vi "log analysis_gps.vi"() -> ()   [LabVIEW 2019] (continued)
11.969600\t-0.937959\t-0.544053\t72.586704\t0.097000\t0.019000\n\t\n15:28:30.8\tlog_raw\tgps_raw\t\tsystem status\texception 0 28.000000 0 60\trobot status\t346.259723\t26.589549\t11.968800\t-0.938206\t-0.546014\t72.587898\t0.097000\t0.019000\n\t\n15:28:31.3\tlog_raw\tgps_raw\t\tsystem status\texception 0 28.100000 0 60\trobot status\t346.261225\t26.595016\t11.967900\t-0.938058\t-0.546498\t72.587416\t0.097000\t0.019000\n\t\n15:28:31.8\tlog_raw\tgps_raw\t\tsystem status\texception 0 28.100000 0 60\trobot status\t346.263217\t26.600750\t11.967200\t-0.937314\t-0.548987\t72.586839\t0.097000\t0.019000\n\t\n15:28:32.3\tlog_raw\tgps_raw\t\tsystem status\texception 0 28.100000 0 60\trobot status\t346.266027\t26.606616\t11.967100\t-0.934688\t-0.548051\t72.585281\t0.097000\t0.019000\n\t\n15:28:32.8\tlog_raw\tgps_raw\t\tsystem status\texception 0 28.000000 0 60\trobot status\t346.269388\t26.612663\t11.967500\t-0.933167\t-0.552134\t72.585486\t0.097000\t0.019000\n\t\n15:28:33.3\tlog_raw\tgps_raw\t\tsystem status\texception 0 28.100000 0 60\trobot status\t346.272370\t26.617656\t11.968500\t-0.933128\t-0.553139\t72.580572\t0.097000\t0.019000\n\t\n15:28:33.8\tlog_raw\tgps_raw\t\tsystem status\texception 0 28.000000 0 60\trobot status\t346.274708\t26.622212\t11.969900\t-0.932001\t-0.554064\t72.578346\t0.097000\t0.019000\n\t\n15:28:34.3\tlog_raw\tgps_raw\t\tsystem status\texception 0 28.000000 0 60\trobot status\t346.272071\t26.616055\t11.970100\t-0.930607\t-0.553691\t72.568592\t0.097000\t0.019000\n\t\n15:28:34.8\tlog_raw\tgps_raw\t#INSPVAXA,USB3,0,50.0,FINESTEERING,2107,282532.800,02000000,471d,15824;INS_ALIGNMENT_COMPLETE,INS_RTKFIXED,37.37036990032,126.72474422565,11.9691,22.3000,0.0075,0.0051,0.0018,-0.932116001,-0.549055451,17.452522918,0.2503,0.2036,0.3279,0.0447,0.0435,0.0399,0.0917,0.0916,4.9913,0f000005,0*47d3a519\n\tsystem status\texception 0 28.000000 0 60\trobot status\t346.263495\t26.596260\t11.969100\t-0.932116\t-0.549055\t72.547477\t0.097000\t0.019000\n\t\n15:28:35.3\tlog_raw\tgps_raw\t\tsystem status\texception 0 28.000000 0 60\trobot status\t346.259446\t26.587060\t11.968800\t-0.932260\t-0.546298\t72.538547\t0.097000\t0.019000\n\t\n15:28:35.8\tlog_raw\tgps_raw\t\tsystem status\texception 0 28.000000 0 60\trobot status\t346.258585\t26.585056\t11.968900\t-0.932112\t-0.548446\t72.536891\t0.097000\t0.019000\n\t\n15:28:36.3\tlog_raw\tgps_raw\t\tsystem status\texception 0 28.000000 0 60\trobot status\t346.258032\t26.583583\t11.969100\t-0.930409\t-0.549639\t72.534290\t0.097000\t0.019000\n\t\n15:28:36.8\tlog_raw\tgps_raw\t\tsystem status\tnormal 0 28.000000 0 0\trobot status\t346.258148\t26.582748\t11.969400\t-0.931772\t-0.548957\t72.530403\t0.000000\t0.000000\n\t\n15:28:37.3\tlog_raw\tgps_raw\t\tsystem status\tnormal 0 28.100000 0 0\trobot status\t346.258252\t26.582082\t11.969800\t-0.931421\t-0.548856\t72.527417\t0.000000\t0.000000\n\t\n15:28:37.8\tlog_raw\tgps_raw\t#INSPVAXA,USB3,0,51.5,FINESTEERING,2107,282535.800,02000000,471d,15824;INS_ALIGNMENT_COMPLETE,INS_RTKFIXED,37.37036976834,126.72474416785,11.9702,22.3000,0.0056,0.0032,0.0025,-0.929895775,-0.548968401,17.475093869,0.2332,0.1853,0.3065,0.0346,0.0344,0.0316,0.0907,0.0908,4.9937,0f000005,0*4023dcd5\n\tsystem status\tnormal 0 28.000000 0 0\trobot status\t346.258376\t26.581613\t11.970200\t-0.929896\t-0.548968\t72.524906\t0.000000\t0.000000\n\t\n15:28:38.3\tlog_raw\tgps_raw\t\tsystem status\tnormal 0 28.100000 0 0\trobot status\t346.258500\t26.581480\t11.970500\t-0.929563\t-0.547939\t72.523200\t0.000000\t0.000000\n\t\n15:28:38.8\tlog_raw\tgps_raw\t\tsystem status\tnormal 0 28.100000 0 0\trobot status\t346.259099\t26.581501\t11.970800\t-0.929146\t-0.547594\t72.520945\t0.000000\t0.000000\n\t\n15:28:39.3\tlog_raw\tgps_raw\t\tsystem status\tnormal 0 28.100000 0 0\trobot status\t346.259649\t26.581507\t11.971100\t-0.930249\t-0.547598\t72.515508\t0.000000\t0.000000\n\t\n15:28:39.8\tlog_raw\tgps_raw\t\tsystem status\tnormal 0 28.000000 0 0\trobot status\t346.260387\t26.581691\t11.971500\t-0.931613\t-0.550759\t72.514164\t0.000000\t0.000000\n\t\n15:28:40.3\tlog_raw\tgps_raw\t\tsystem status\tnormal 0 28.000000 0 0\trobot status\t346.261018\t26.582062\t11.972200\t-0.929740\t-0.553791\t72.508433\t0.000000\t0.000000\n\t\n15:28:40.8\tlog_raw\tgps_raw\t\tsystem status\tnormal 0 28.100000 0 0\trobot status\t346.261462\t26.582894\t11.973100\t-0.928845\t-0.555133\t72.506321\t0.000000\t0.000000\n\t\n15:28:41.3\tlog_raw\tgps_raw\t#INSPVAXA,USB3,0,50.0,FINESTEERING,2107,282539.300,02000000,471d,15824;INS_ALIGNMENT_COMPLETE,INS_RTKFIXED,37.37036978494,126.72474420325,11.9738,22.3000,0.0064,0.0050,0.0000,-0.929010849,-0.553956795,17.498282096,0.2195,0.1742,0.2911,0.0344,0.0343,0.0312,0.0907,0.0907,4.9970,0f000005,0*d5ca5fec\n\tsystem status\tnormal 0 28.000000 0 0\trobot status\t346.261511\t26.583455\t11.973800\t-0.929011\t-0.553957\t72.501718\t0.000000\t0.000000\n\t\n15:28:41.8\tlog_raw\tgps_raw\t#INSPVAXA,USB3,0,50.0,FINESTEERING,2107,282539.800,02000000,471d,15824;INS_ALIGNMENT_COMPLETE,INS_RTKFIXED,37.37036978547,126.72474420294,11.9740,22.3000,0.0057,0.0046,-0.0006,-0.928135353,-0.553814797,17.500957060,0.2195,0.1742,0.2911,0.0344,0.0343,0.0312,0.0907,0.0907,4.9970,0f000005,0*764a2b63\n\tsystem status\tnormal 0 28.000000 0 0\trobot status\t346.261484\t26.583514\t11.974000\t-0.928135\t-0.553815\t72.499043\t0.000000\t0.000000\n\t\n15:28:42.3\tlog_raw\tgps_raw\t\tsystem status\tnormal 0 28.100000 0 0\trobot status\t346.261404\t26.583443\t11.974300\t-0.930384\t-0.553797\t72.496316\t0.000000\t0.000000\n\t\n15:28:42.8\tlog_raw\tgps_raw\t#INSPVAXA,USB3,0,51.5,FINESTEERING,2107,282540.800,02000000,471d,15824;INS_ALIGNMENT_COMPLETE,INS_RTKFIXED,37.37036978786,126.72474420160,11.9749,22.3000,0.0059,0.0033,-0.0010,-0.930808234,-0.552950862,17.507619402,0.2170,0.1726,0.2881,0.0344,0.0343,0.0312,0.0907,0.0907,4.9979,0f000005,0*a62a7559\n\tsystem status\tnormal 0 28.100000 0 0\trobot status\t346.261365\t26.583779\t11.974900\t-0.930808\t-0.552951\t72.492381\t0.000000\t0.000000\n\t\n15:28:43.3\tlog_raw\tgps_raw\t#INSPVAXA,USB3,0,52.0,FINESTEERING,2107,282541.300,02000000,471d,15824;INS_ALIGNMENT_COMPLETE,INS_RTKFIXED,37.37036978965,126.72474419874,11.9755,22.3000,0.0062,0.0033,-0.0009,-0.929974258,-0.549981203,17.509762902,0.2148,0.1713,0.2853,0.0344,0.0343,0.0312,0.0907,0.0906,4.9990,0f000005,0*bfdf10fc\n\tsystem status\tnormal 0 28.000000 0 0\trobot status\t346.261112\t26.583978\t11.975500\t-0.929974\t-0.549981\t72.490237\t0.000000\t0.000000\n\t\n15:28:43.8\tlog_raw\tgps_raw\t\tsystem status\tnormal 0 28.100000 0 0\trobot status\t346.261132\t26.584205\t11.975800\t-0.930744\t-0.550329\t72.489076\t0.000000\t0.000000\n\t\n15:28:44.3\tlog_raw\tgps_raw\t#INSPVAXA,USB3,0,51.0,FINESTEERING,2107,282542.300,02000000,471d,15824;INS_ALIGNMENT_COMPLETE,INS_RTKFIXED,37.37036979234,126.72474420075,11.9765,22.3000,0.0055,0.0042,-0.0011,-0.931303287,-0.550383804,17.513004311,0.2130,0.1703,0.2828,0.0344,0.0343,0.0312,0.0907,0.0906,5.0000,0f000005,0*b690bd46\n\tsystem status\tnormal 0 28.000000 0 0\trobot status\t346.261290\t26.584276\t11.976500\t-0.931303\t-0.550384\t72.486996\t0.000000\t0.000000\n\t\n15:28:44.8\tlog_raw\tgps_raw\t\tsystem status\tnormal 0 28.000000 0 0\trobot status\t346.261465\t26.584112\t11.977300\t-0.929492\t-0.551225\t72.486272\t0.000000\t0.000000\n\t\n15:28:45.3\tlog_raw\tgps_raw\t#INSPVAXA,USB3,0,47.5,FINESTEERING,2107,282543.300,02000000,471d,15824;INS_ALIGNMENT_COMPLETE,INS_RTKFIXED,37.37036978809,126.72474420745,11.9781,22.3000,0.0036,0.0055,-0.0013,-0.931308273,-0.552026668,17.515229582,0.2114,0.1694,0.2805,0.0344,0.0343,0.0312,0.0907,0.0906,5.0009,0f000005,0*ba0ef0aa\n\tsystem status\tnormal 0 28.000000 0 0\trobot status\t346.261883\t26.583805\t11.978100\t-0.931308\t-0.552027\t72.484770\t0.000000\t0.000000\n\t\n15:28:45.8\tlog_raw\tgps_raw\t#INSPVAXA,USB3,0,47.5,FINESTEERING,2107,282543.800,02000000,471d,15824;INS_ALIGNMENT_COMPLETE,INS_RTKFIXED,37.37036978808,126.72474421663,11.9786,22.3000,0.0047,0.0067,-0.0013,-0.928872282,-0.553697903,17.517066797,0.2114,0.1694,0.2805,0.0344,0.0343,0.0312,0.0907,0.0906,5.0009,0f000005,0*82370f01\n\tsystem status\tnormal 0 28.100000 0 0\trobot status\t346.262696\t26.583804\t11.978600\t-0.928872\t-0.553698\t72.482933\t0.000000\t0.000000\n\t\n15:28:46.3\tlog_raw\tgps_raw\t#INSPVAXA,USB3,0,48.0,FINESTEERING,2107,282544.300,02000000,471d,15824;INS_ALIGNMENT_COMPLETE,INS_RTKFIXED,37.37036978718,126.72474422252,11.9791,22.3000,0.0050,0.0075,-0.0009,-0.927752537,-0.554071617,17.520424988,0.2100,0.1688,0.2784,0.0344,0.0343,0.0312,0.0907,0.0906,5.0016,0f000005,0*49ddb25e\n\tsystem status\tnormal 0 28.100000 0 0\trobot status\t346.263218\t26.583704\t11.979100\t-0.927753\t-0.554072\t72.479575\t0.000000\t0.000000\n\t\n15:28:46.8\tlog_raw\tgps_raw\t\tsystem status\tnormal 0 28.100000 0 0\trobot status\t346.263972\t26.583698\t11.979500\t-0.928560\t-0.556020\t72.475289\t0.000000\t0.000000\n\t\n15:28:47.3\tlog_raw\tgps_raw\t#INSPVAXA,USB3,0,53.5,FINESTEERING,2107,282545.300,02000000,471d,15824;INS_ALIGNMENT_COMPLETE,INS_RTKFIXED,37.37036978780,126.72474423597,11.9800,22.3000,0.0057,0.0083,-0.0009,-0.928955270,-0.556659183,17.532369164,0.2088,0.1684,0.2765,0.0344,0.0343,0.0312,0.0907,0.0906,5.0023,0f000005,0*6d6cecb2\n\tsystem status\tnormal 0 28.100000 0 0\trobot status\t346.264409\t26.583772\t11.980000\t-0.928955\t-0.556659\t72.467631\t0.000000\t0.000000\n\t\n15:28:47.8\tlog_raw\tgps_raw\t#INSPVAXA,USB3,0,53.5,FINESTEERING,2107,282545.800,02000000,471d,15824;INS_ALIGNMENT_COMPLETE,INS_RTKFIXED,37.37036979074,126.72474423499,11.9811,22.3000,0.0059,0.0071,-0.0001,-0.929937499,-0.555084001,17.534967514,0.2088,0.1684,0.2765,0.0344,0.0343,0.0312,0.0907,0.0906,5.0023,0f000005,0*3f4b51d6\n\tsystem status\tnormal 0 28.000000 0 0\trobot status\t346.264323\t26.584099\t11.981100\t-0.929937\t-0.555084\t72.465032\t0.000000\t0.000000\n\t\n15:28:48.3\tlog_raw\tgps_raw\t#INSPVAXA,USB3,0,52.0,FINESTEERING,2107,282546.300,02000000,471d,15824;INS_ALIGNMENT_COMPLETE,INS_RTKFIXED,37.37036979075,126.72474423167,11.9818,22.3000,0.0060,0.0065,0.0000,-0.930882375,-0.556370443,17.539693499,0.2078,0.1680,0.2748,0.0344,0.0343,0.0312,0.0907,0.0906,5.0033,0f000005,0*966ea92a\n\tsystem status\tnormal 0 28.100000 0 0\trobot status\t346.264029\t26.584100\t11.981800\t-0.930882\t-0.556370\t72.460307\t0.000000\t0.000000\n\t\n15:28:48.8\tlog_raw\tgps_raw\t#INSPVAXA,USB3,0,52.0,FINESTEERING,2107,282546.800,02000000,471d,15824;INS_ALIGNMENT_COMPLETE,INS_RTKFIXED,37.37036979117,126.72474423599,11.9822,22.3000,0.0059,0.0073,0.0004,-0.930733937,-0.558015059,17.542914656,0.2078,0.1680,0.2748,0.0344,0.0343,0.0312,0.0907,0.0906,5.0033,0f000005,0*c41d3119\n\tsystem status\tnormal 0 28.000000 0 0\trobot status\t346.264411\t26.584146\t11.982200\t-0.930734\t-0.558015\t72.457085\t0.000000\t0.000000\n\t\n15:28:49.3\tlog_raw\tgps_raw\t#INSPVAXA,USB3,0,48.0,FINESTEERING,2107,282547.300,02000000,471d,15824;INS_ALIGNMENT_COMPLETE,INS_RTKFIXED,37.37036978952,126.72474423883,11.9826,22.3000,0.0057,0.0074,0.0003,-0.934085906,-0.556515155,17.545794834,0.2070,0.1677,0.2732,0.0344,0.0343,0.0312,0.0907,0.0906,5.0042,0f000005,0*0a93c56e\n\tsystem status\tnormal 0 28.000000 0 0\trobot status\t346.264663\t26.583963\t11.982600\t-0.934086\t-0.556515\t72.454205\t0.000000\t0.000000\n\t\n15:28:49.8\tlog_raw\tgps_raw\t#INSPVAXA,USB3,0,48.0,FINESTEERING,2107,282547.800,02000000,471d,15824;INS_ALIGNMENT_COMPLETE,INS_RTKFIXED,37.37036979022,126.72474424169,11.9829,22.3000,0.0059,0.0077,0.0009,-0.935404379,-0.556069366,17.549298346,0.2070,0.1677,0.2732,0.0344,0.0343,0.0312,0.0907,0.0906,5.0042,0f000005,0*a5f569c8\n\tsystem status\tnormal 0 28.100000 0 0\trobot status\t346.264916\t26.584041\t11.982900\t-0.935404\t-0.556069\t72.450702\t0.000000\t0.000000\n\t\n15:28:50.3\tlog_raw\tgps_raw\t#INSPVAXA,USB3,0,52.0,FINESTEERING,2107,282548.300,02000000,471d,15824;INS_ALIGNMENT_COMPLETE,INS_RTKFIXED,37.37036979009,126.72474424298,11.9833,22.3000,0.0058,0.0072,0.0008,-0.938145117,-0.556054082,17.551756735,0.2062,0.1674,0.2718,0.0344,0.0343,0.0312,0.0907,0.0906,5.0051,0f000005,0*c2e33c02\n\tsystem status\tnormal 0 28.100000 0 0\trobot status\t346.265030\t26.584027\t11.983300\t-0.938145\t-0.556054\t72.448243\t0.000000\t0.000000\n\t\n15:28:50.8\tlog_raw\tgps_raw\t\tsystem status\tnormal 0 28.100000 0 0\trobot status\t346.265084\t26.584261\t11.983800\t-0.940336\t-0.557104\t72.445963\t0.000000\t0.000000\n\t\n15:28:51.3\tlog_raw\tgps_raw\t#INSPVAXA,USB3,0,50.5,FINESTEERING,2107,282549.300,02000000,471d,15824;INS_ALIGNMENT_COMPLETE,INS_RTKFIXED,37.37036979437,126.72474424171,11.9842,22.3000,0.0072,0.0058,0.0011,-0.941172709,-0.557765925,17.557830544,0.2056,0.1673,0.2705,0.0344,0.0343,0.0312,0.0907,0.0905,5.0063,0f000005,0*401534f2\n\tsystem status\tnormal 0 28.100000 0 0\trobot status\t346.264918\t26.584502\t11.984200\t-0.941173\t-0.557766\t72.442169\t0.000000\t0.000000\n\t\n15:28:51.8\tlog_raw\tgps_raw\t#INSPVAXA,USB3,0,50.5,FINESTEERING,2107,282549.800,02000000,471d,15824;INS_ALIGNMENT_COMPLETE,INS_RTKFIXED,37.37037057498,126.72474454669,11.9842,22.3000,0.3344,0.1212,-0.0021,-0.779908756,-0.829652021,16.234479944,0.2056,0.1673,0.2705,0.0344,0.0343,0.0312,0.0907,0.0905,5.0063,0f000005,0*992e23a9\n\tsystem status\tnormal 2 27.900000 0 0\trobot status\t346.291933\t26.671136\t11.984200\t-0.779909\t-0.829652\t73.765520\t0.366000\t0.090000\n\t\n15:28:52.3\tlog_raw\tgps_raw\t#INSPVAXA,USB3,0,48.5,FINESTEERING,2107,282550.300,02000000,471d,15824;INS_ALIGNMENT_COMPLETE,INS_RTKFIXED,37.37037180552,126.72474490570,11.9839,22.3000,0.3136,0.0717,0.0047,-0.762896217,-1.138555506,11.977754851,0.2091,0.1720,0.2750,0.0478,0.0529,0.0400,0.0942,0.0940,5.0079,0f000001,0*abd47146\n\tsystem status\tnormal 2 27.200000 0 0\trobot status\t346.323733\t26.807706\t11.983900\t-0.762896\t-1.138556\t78.022245\t0.332000\t0.113000\n\t\n15:28:52.8\tlog_raw\tgps_raw\t#INSPVAXA,USB3,0,48.5,FINESTEERING,2107,282550.800,02000000,471d,15824;INS_ALIGNMENT_COMPLETE,INS_RTKFIXED,37.37037314462,126.72474521124,11.9825,22.3000,0.2954,0.0405,-0.0041,-0.725905831,-1.406758813,6.746591451,0.2091,0.1720,0.2750,0.0478,0.0529,0.0400,0.0942,0.0940,5.0079,0f000001,0*61668905\n\tsystem status\tnormal 2 27.200000 4 0\trobot status\t346.350797\t26.956324\t11.982500\t-0.725906\t-1.406759\t83.253409\t0.297000\t0.188000\n\t\n15:28:53.3\tlog_raw\tgps_raw\t#INSPVAXA,USB3,0,51.5,FINESTEERING,2107,282551.300,02000000,471d,15824;INS_ALIGNMENT_COMPLETE,INS_RTKFIXED,37.37037450282,126.72474542954,11.9799,22.3000,0.2952,0.0275,0.0043,-0.582539496,-1.551817939,1.239321391,0.2194,0.1781,0.2846,0.0602,0.0670,0.0471,0.0975,0.0974,5.0042,0f000001,0*c43f8c5d\n\tsystem status\tnormal 2 27.300000 4 0\trobot status\t346.370134\t27.107063\t11.979900\t-0.582539\t-1.551818\t88.760679\t0.286000\t0.198000\n\t\n15:28:53.8\tlog_raw\tgps_raw\t#INSPVAXA,USB3,0,51.5,FINESTEERING,2107,282551.800,02000000,471d,15824;INS_ALIGNMENT_COMPLETE,INS_RTKFIXED,37.37037589392,126.72474545445,11.9759,22.3000,0.2950,0.0095,-0.0088,-0.557235878,-1.675921373,356.051789382,0.2194,0.1781,0.2846,0.0602,0.0670,0.0471,0.0975,0.0974,5.0042,0f000001,0*a284eeef\n\tsystem status\tnormal 2 27.300000 4 0\trobot status\t346.372340\t27.261453\t11.975900\t-0.557236\t-1.675921\t93.948211\t0.253000\t0.253000\n\t\n15:28:54.3\tlog_raw\tgps_raw\t#INSPVAXA,USB3,0,51.0,FINESTEERING,2107,282552.300,02000000,471d,15824;INS_ALIGNMENT_COMPLETE,INS_RTKFIXED,37.37037725637,126.72474539414,11.9729,22.3000,0.3193,-0.0395,-0.0058,-0.358098572,-1.586037546,351.118490428,0.2390,0.1944,0.2996,0.0720,0.0761,0.0531,0.1006,0.1005,4.9843,0f000001,0*9b67c117\n\tsystem status\tnormal 2 27.200000 0 0\trobot status\t346.366998\t27.412664\t11.972900\t-0.358099\t-1.586038\t98.881510\t0.274000\t0.215000\n\t\n15:28:54.8\tlog_raw\tgps_raw\t#INSPVAXA,USB3,0,51.0,FINESTEERING,2107,282552.800,02000000,471d,15824;INS_ALIGNMENT_COMPLETE,INS_RTKFIXED,37.37037867024,126.72474521498,11.9693,22.3000,0.3100,-0.0524,0.0074,-0.558642327,-1.723684038,345.940999200,0.2390,0.1944,0.2996,0.0720,0.0761,0.0531,0.1006,0.1005,4.9843,0f000001,0*b237e03e\n\tsystem status\tnormal 2 27.200000 0 0\trobot status\t346.351129\t27.569583\t11.969300\t-0.558642\t-1.723684\t104.059001\t0.330000\t0.150000\n\t\n15:28:55.3\tlog_raw\tgps_raw\t\tsystem status\tnormal 2 27.300000 4 0\trobot status\t346.324168\t27.702599\t11.965400\t-0.427225\t-1.756505\t108.753791\t0.296000\t0.197000\n\t\n15:28:55.8\tlog_raw\tgps_raw\t#INSPVAXA,USB3,0,50.0,FINESTEERING,2107,282553.800,02000000,471d,15824;INS_ALIGNMENT_COMPLETE,INS_RTKFIXED,37.37038133440,126.72474444492,11.9605,22.3000,0.3081,-0.0778,-0.0137,-0.440969194,-1.715960461,335.579383056,0.2674,0.2182,0.3198,0.0835,0.0827,0.0582,0.1031,0.1033,4.9481,0f000001,0*e6869deb\n\tsystem status\tnormal 2 27.200000 0 0\trobot status\t346.282918\t27.865266\t11.960500\t-0.440969\t-1.715960\t114.420617\t0.345000\t0.173000\n\t\n15:28:56.3\tlog_raw\tgps_raw\t#INSPVAXA,USB3,0,50.5,FINESTEERING,2107,282554.300,02000000,471d,15824;INS_ALIGNMENT_COMPLETE,INS_RTKFIXED,37.37038260490,126.72474387942,11.9550,22.3000,0.2856,-0.1157,-0.0141,-0.305818210,-1.684904810,330.613449941,0.3015,0.2424,0.3440,0.0942,0.0885,0.0625,0.1050,0.1055,4.9097,0f000001,0*224ecce4\n\tsystem status\tnormal 2 27.200000 4 0\trobot status\t346.232827\t28.006274\t11.955000\t-0.305818\t-1.684905\t119.386550\t0.285000\t0.202000\n\t\n15:28:56.8\tlog_raw\tgps_raw\t#INSPVAXA,USB3,0,50.5,FINESTEERING,2107,282554.800,02000000,471d,15824;INS_ALIGNMENT_COMPLETE,INS_RTKFIXED,37.37038381003,126.72474321955,11.9506,22.3000,0.2827,-0.1438,-0.0083,-0.269920364,-1.529846026,325.201495362,0.3015,0.2424,0.3440,0.0942,0.0885,0.0625,0.1050,0.1055,4.9097,0f000001,0*3a829f91\n\tsystem status\tnormal 2 27.300000 4 0\trobot status\t346.174377\t28.140028\t11.950600\t-0.269920\t-1.529846\t124.798505\t0.313000\t0.169000\n\t\n15:28:57.3\tlog_raw\tgps_raw\t#INSPVAXA,USB3,0,50.0,FINESTEERING,2107,282555.300,02000000,471d,15824;INS_ALIGNMENT_COMPLETE,INS_RTKFIXED,37.37038496801,126.72474241807,11.9455,22.3000,0.2577,-0.2027,-0.0062,-0.202108415,-1.553117740,320.165911198,0.3366,0.2625,0.3706,0.1033,0.0925,0.0661,0.1060,0.1070,4.8793,0f000001,0*992111cd\n\tsystem status\tnormal 2 27.200000 4 0\trobot status\t346.103383\t28.268549\t11.945500\t-0.202108\t-1.553118\t129.834089\t0.289000\t0.205000\n\t\n15:28:57.8\tlog_raw\tgps_raw\t#INSPVAXA,USB3,0,50.0,FINESTEERING,2107,282555.800,02000000,471d,15824;INS_ALIGNMENT_COMPLETE,INS_RTKFIXED,37.37038604879,126.72474155018,11.9405,22.3000,0.2577,-0.1938,-0.0290,0.085654909,-1.443333237,315.847452046,0.3366,0.2625,0.3706,0.1033,0.0925,0.0661,0.1060,0.1070,4.8793,0f000001,0*a6375ebe\n\tsystem status\tnormal 2 27.300000 4 0\trobot status\t346.026507\t28.388502\t11.940500\t0.085655\t-1.443333\t134.152548\t0.303000\t0.148000\n\t\n15:28:58.3\tlog_raw\tgps_raw\t#INSPVAXA,USB3,0,47.0,FINESTEERING,2107,282556.300,02000000,471d,15824;INS_ALIGNMENT_COMPLETE,INS_RTKFIXED,37.37038704857,126.72474062241,11.9355,22.3000,0.2432,-0.1774,-0.0062,0.142331168,-1.481321498,311.639962663,0.3685,0.2772,0.3979,0.1103,0.0957,0.0690,0.1063,0.1076,4.8620,0f000001,0*be30efa1\n\tsystem status\tnormal 2 27.300000 4 0\trobot status\t345.944326\t28.499465\t11.935500\t0.142331\t-1.481321\t138.360037\t0.292000\t0.150000\n\t\n15:28:58.8\tlog_raw\tgps_raw\t#INSPVAXA,USB3,0,47.0,FINESTEERING,2107,282556.800,02000000,471d,15824;INS_ALIGNMENT_COMPLETE,INS_RTKFIXED,37.37038792888,126.72473964017,11.9328,22.3000,0.2236,-0.2049,0.0022,0.167042140,-1.399079221,308.149842307,0.3685,0.2772,0.3979,0.1103,0.0957,0.0690,0.1063,0.1076,4.8620,0f000001,0*295fc098\n\tsystem status\tnormal 2 27.300000 4 0\trobot status\t345.857321\t28.597170\t11.932800\t0.167042\t-1.399079\t141.850158\t0.297000\t0.135000\n\t\n15:28:59.3\tlog_raw\tgps_raw\t#INSPVAXA,USB3,0,49.5,FINESTEERING,2107,282557.300,02000000,471d,15824;INS_ALIGNMENT_COMPLETE,INS_RTKFIXED,37.37038876743,126.72473857634,11.9284,22.3000,0.2199,-0.2115,-0.0007,0.223675096,-1.209289977,305.425052983,0.3945,0.2871,0.4244,0.1154,0.0985,0.0713,0.1059,0.1076,4.8550,0f000001,0*37184781\n\tsystem status\tnormal 2 27.300000 4 0\trobot status\t345.763089\t28.690240\t11.928400\t0.223675\t-1.209290\t144.574947\t0.319000\t0.054000\n\t\n15:28:59.8\tlog_raw\tgps_raw\t#INSPVAXA,USB3,0,49.5,FINESTEERING,2107,282557.800,02000000,471d,15824;INS_ALIGNMENT_COMPLETE,INS_RTKFIXED,37.37038956876,126.72473745081,11.9243,22.3000,0.2096,-0.2177,-0.0233,0.358750528,-1.202788361,303.229385124,0.3945,0.2871,0.4244,0.1154,0.0985,0.0713,0.1059,0.1076,4.8550,0f000001,0*8c1e375a\n\tsystem status\tnormal 2 27.400000 4 0\trobot status\t345.663391\t28.779179\t11.924300\t0.358751\t-1.202788\t146.770615\t0.305000\t0.061000\n\t\n15:29:00.3\tlog_raw\tgps_raw\t#INSPVAXA,USB3,0,50.5,FINESTEERING,2107,282558.300,02000000,471d,15824;INS_ALIGNMENT_COMPLETE,INS_RTKFIXED,37.37039033864,126.72473628263,11.9208,22.3000,0.2004,-0.2164,-0.0069,0.499556511,-1.306604746,301.526266622,0.4138,0.2933,0.4487,0.1187,0.1006,0.0729,0.1051,0.1069,4.8540,0f000001,0*451656bf\n\tsystem status\tnormal 2 27.500000 4 0\trobot status\t345.559916\t28.864628\t11.920800\t0.499557\t-1.306605\t148.473733\t0.303000\t0.041000\n\t\n15:29:00.8\tlog_raw\tgps_raw\t#INSPVAXA,USB3,0,50.5,FINESTEERING,2107,282558.800,02000000,471d,15824;INS_ALIGNMENT_COMPLETE,INS_RTKFIXED,37.37039107336,126.72473508379,11.9182,22.3000,0.1823,-0.2245,-0.0036,0.428634950,-1.459936721,300.166492995,0.4138,0.2933,0.4487,0.1187,0.1006,0.0729,0.1051,0.1069,4.8540,0f000001,0*b88ea368\n\tsystem status\tnormal 2 27.600000 0 0\trobot status\t345.453724\t28.946175\t11.918200\t0.428635\t-1.459937\t149.833507\t0.302000\t0.033000\n\t\n15:29:01.3\tlog_raw\tgps_raw\t#INSPVAXA,USB3,0,48.0,FINESTEERING,2107,282559.300,02000000,471d,15824;INS_ALIGNMENT_COMPLETE,INS_RTKFIXED,37.37039179926,126.72473381878,11.9163,22.3000,0.1950,-0.2202,-0.0095,0.298148012,-1.385671812,299.213023137,0.4272,0.2974,0.4700,0.1208,0.1020,0.0740,0.1041,0.1060,4.8546,0f000001,0*f3b6d2c4\n\tsystem status\tnormal 2 27.700000 0 0\trobot status\t345.341672\t29.026744\t11.916300\t0.298148\t-1.385672\t150.786977\t0.246000\t0.117000\n\t\n15:29:01.8\tlog_raw\tgps_raw\t#INSPVAXA,USB3,0,48.0,FINESTEERING,2107,282559.800,02000000,471d,15824;INS_ALIGNMENT_COMPLETE,INS_RTKFIXED,37.37039251718,126.72473255012,11.9132,22.3000,0.1990,-0.2202,-0.0184,0.279170037,-1.304746130,298.607357050,0.4272,0.2974,0.4700,0.1208,0.1020,0.0740,0.1041,0.1060,4.8546,0f000001,0*fce9781a\n\tsystem status\tnormal 2 27.800000 0 0\trobot status\t345.229296\t29.106426\t11.913200\t0.279170\t-1.304746\t151.392643\t0.262000\t0.089000\n\t\n15:29:02.3\tlog_raw\tgps_raw\t#DUALANTENNAHEADINGA,USB3,0,49.0,FINESTEERING,2107,282560.300,02000000,d426,15824;SOL_COMPUTED,L1_FLOAT,-1.000000000,246.253692627,40.984443665,0.0,360.000000000,180.000000000,\"631T\",16,4,4,4,04,00,20,00*676df0ad\n\tsystem status\tnormal 2 27.900000 0 0\trobot status\t345.113905\t29.186106\t11.908100\t0.286139\t-1.166642\t151.713983\t0.238000\t0.100000\n\t\n15:29:02.8\tlog_raw\tgps_raw\t#INSPVAXA,USB3,0,49.0,FINESTEERING,2107,282560.800,02000000,471d,15824;INS_ALIGNMENT_COMPLETE,INS_RTKFIXED,37.37039395485,126.72472993141,11.9024,22.3000,0.2031,-0.2330,-0.0176,0.316707422,-1.216731962,298.161405387,0.4358,0.3002,0.4880,0.1220,0.1029,0.0748,0.1029,0.1049,4.8545,0f000001,0*df5ab1e4\n\tsystem status\tnormal 2 27.900000 0 0\trobot status\t344.997335\t29.265995\t11.902400\t0.316707\t-1.216732\t151.838595\t0.288000\t0.019000\n\t\n15:29:03.3\tlog_raw\tgps_raw\t#DUALANTENNAHEADINGA,USB3,0,50.5,FINESTEERING,2107,282561.300,02000000,d426,15824;SOL_COMPUTED,L1_FLOAT,-1.000000000,334.919982910,-70.914154053,0.0,360.000000000,180.000000000,\"631T\",14,4,4,4,04,00,20,00*464ca699\n\tsystem status\tnormal 2 27.900000 0 0\trobot status\t344.878996\t29.343768\t11.898300\t0.167702\t-1.243399\t151.906348\t0.328000\t-0.042000\n\t\n15:29:03.8\tlog_raw\tgps_raw\t#INSPVAXA,USB3,0,50.5,FINESTEERING,2107,282561.800,02000000,471d,15824;INS_ALIGNMENT_COMPLETE,INS_RTKFIXED,37.37039536755,126.72472721872,11.8937,22.3000,0.2015,-0.2233,-0.0217,0.095358091,-1.276712032,298.220729276,0.4412,0.3019,0.5026,0.1224,0.1030,0.0752,0.1017,0.1038,4.8530,0f000001,0*c4564f75\n\tsystem status\tnormal 2 28.000000 0 0\trobot status\t344.757049\t29.422793\t11.893700\t0.095358\t-1.276712\t151.779271\t0.355000\t-0.097000\n\t\n15:29:04.3\tlog_raw\tgps_raw\t#DUALANTENNAHEADINGA,USB3,0,50.0,FINESTEERING,2107,282562.300,02000000,d426,15824;SOL_COMPUTED,L1_FLOAT,-1.000000000,248.535232544,17.692501068,0.0,360.000000000,180.000000000,\"631T\",15,4,4,4,04,00,20,00*bc5c3482\n\tsystem status\tnormal 2 28.000000 0 0\trobot status\t344.636634\t29.501493\t11.889200\t0.216605\t-1.242844\t151.713367\t0.346000\t-0.081000\n\t\n15:29:04.8\tlog_raw\tgps_raw\t#INSPVAXA,USB3,0,50.0,FINESTEERING,2107,282562.800,02000000,471d,15824;INS_ALIGNMENT_COMPLETE,INS_RTKFIXED,37.37039678441,126.72472449457,11.8837,22.3000,0.2087,-0.2358,-0.0215,0.255454294,-1.083158063,298.402079920,0.4444,0.3029,0.5140,0.1223,0.1022,0.0754,0.1006,0.1028,4.8501,0f000001,0*9eae090a\n\tsystem status\tnormal 2 28.000000 0 0\trobot status\t344.515749\t29.580053\t11.883700\t0.255454\t-1.083158\t151.597920\t0.298000\t-0.001000\n\t\n15:29:05.3\tlog_raw\tgps_raw\t#DUALANTENNAHEADINGA,USB3,0,51.0,FINESTEERING,2107,282563.300,02000000,d426,15824;SOL_COMPUTED,L1_FLOAT,-1.000000000,237.849975586,47.216407776,0.0,360.000000000,180.000000000,\"631T\",15,4,4,4,04,00,20,00*b09d8761\n\tsystem status\tnormal 2 28.000000 0 0\trobot status\t344.396553\t29.657849\t11.878700\t0.203680\t-1.083027\t151.443987\t0.293000\t-0.011000\n\t\n15:29:05.8\tlog_raw\tgps_raw\t#DUALANTENNAHEADINGA,USB3,0,51.0,FINESTEERING,2107,282563.800,02000000,d426,15824;SOL_COMPUTED,L1_FLOAT,-1.000000000,239.350723267,46.591415405,0.0,360.000000000,180.000000000,\"631T\",14,4,4,4,04,00,20,00*f242e7bf\n\tsystem status\tnormal 2 28.000000 0 0\trobot status\t344.272001\t29.740455\t11.874400\t0.239791\t-1.172717\t151.332687\t0.302000\t-0.010000\n\t\n15:29:06.3\tlog_raw\tgps_raw\t#DUALANTENNAHEADINGA,USB3,0,51.0,FINESTEERING,2107,282564.300,02000000,d426,15824;SOL_COMPUTED,L1_FLOAT,-1.000000000,238.787353516,46.982643127,0.0,360.000000000,180.000000000,\"631T\",14,4,4,4,04,00,20,00*054ac6ab\n\tsystem status\tnormal 2 28.000000 0 0\trobot status\t344.152987\t29.820091\t11.871500\t0.282375\t-1.336800\t151.200534\t0.300000\t-0.014000\n\t\n15:29:06.8\tlog_raw\tgps_raw\t#DUALANTENNAHEADINGA,USB3,0,51.0,FINESTEERING,2107,282564.800,02000000,d426,15824;SOL_COMPUTED,L1_FLOAT,-1.000000000,245.656951904,39.742870331,0.0,360.000000000,180.000000000,\"631T\",14,4,4,4,04,00,20,00*f11cb885\n\tsystem status\tnormal 2 28.000000 0 0\trobot status\t344.030863\t29.902547\t11.869300\t0.345111\t-1.545641\t151.065776\t0.302000\t-0.011000\n\t\n15:29:07.3\tlog_raw\tgps_raw\t#DUALANTENNAHEADINGA,USB3,0,52.0,FINESTEERING,2107,282565.300,02000000,d426,15824;SOL_COMPUTED,L1_FLOAT,-1.000000000,248.154891968,40.657573700,0.0,360.000000000,180.000000000,\"631T\",14,4,4,4,04,00,20,00*20192c08\n\tsystem status\tnormal 2 28.000000 0 0\trobot status\t343.908952\t29.984892\t11.866600\t0.424566\t-1.614157\t150.906237\t0.299000\t-0.008000\n\t\n15:29:07.8\tlog_raw\tgps_raw\t#INSPVAXA,USB3,0,52.0,FINESTEERING,2107,282565.800,02000000,471d,15824;INS_ALIGNMENT_COMPLETE,INS_RTKFIXED,37.37040119345,126.72471623377,11.8630,22.3000,0.2075,-0.2604,-0.0264,0.476736901,-1.637367273,299.264508322,0.4468,0.3026,0.5333,0.1200,0.0984,0.0755,0.0985,0.1009,4.8387,0f000001,0*ff25f4bc\n\tsystem status\tnormal 2 28.000000 0 0\trobot status\t343.784020\t30.069418\t11.863000\t0.476737\t-1.637367\t150.735492\t0.299000\t-0.008000\n\t\n15:29:08.3\tlog_raw\tgps_raw\t#INSPVAXA,USB3,0,51.5,FINESTEERING,2107,282566.300,02000000,471d,15824;INS_ALIGNMENT_COMPLETE,INS_RTKFIXED,37.37040195558,126.72471483727,11.8592,22.3000,0.1958,-0.2436,-0.0278,0.510354865,-1.544191392,299.414254294,0.4462,0.3017,0.5364,0.1190,0.0970,0.0755,0.0983,0.1007,4.8363,0f000001,0*b461588d\n\tsystem status\tnormal 2 28.000000 0 0\trobot status\t343.660321\t30.154008\t11.859200\t0.510355\t-1.544191\t150.585746\t0.300000\t0.000000\n\t\n15:29:08.8\tlog_raw\tgps_raw\t#INSPVAXA,USB3,0,51.5,FINESTEERING,2107,282566.800,02000000,471d,15824;INS_ALIGNMENT_COMPLETE,INS_RTKFIXED,37.37040269281,126.72471352564,11.8555,22.3000,0.1908,-0.2417,-0.0283,0.566870659,-1.494613883,299.549327154,0.4462,0.3017,0.5364,0.1190,0.0970,0.0755,0.0983,0.1007,4.8363,0f000001,0*0dca09ad\n\tsystem status\tnormal 2 28.000000 0 0\trobot status\t343.544139\t30.235834\t11.855500\t0.566871\t-1.494614\t150.450673\t0.296000\t0.000000\n\t\n15:29:09.3\tlog_raw\tgps_raw\t#DUALANTENNAHEADINGA,USB3,0,48.5,FINESTEERING,2107,282567.300,02000000,d426,15824;SOL_COMPUTED,L1_FLOAT,-1.000000000,255.600921631,36.764995575,0.0,360.000000000,180.000000000,\"631T\",14,4,4,4,04,00,20,00*5c98ac44\n\tsystem status\tnormal 2 28.000000 0 0\trobot status\t343.417441\t30.324121\t11.850100\t0.603379\t-1.447591\t150.332757\t0.306000\t-0.006000\n\t\n15:29:09.8\tlog_raw\tgps_raw\t#DUALANTENNAHEADINGA,USB3,0,48.5,FINESTEERING,2107,282567.800,02000000,d426,15824;SOL_COMPUTED,L1_FLOAT,-1.000000000,256.974517822,34.665092468,0.0,360.000000000,180.000000000,\"631T\",13,4,4,4,04,00,20,00*958b7579\n\tsystem status\tnormal 2 28.000000 0 0\trobot status\t343.297973\t30.408828\t11.845400\t0.569313\t-1.557753\t150.273746\t0.300000\t0.006000\n\t\n15:29:10.3\tlog_raw\tgps_raw\t#DUALANTENNAHEADINGA,USB3,0,47.5,FINESTEERING,2107,282568.300,02000000,d426,15824;SOL_COMPUTED,L1_FLOAT,-1.000000000,267.947265625,0.986307323,0.0,360.000000000,180.000000000,\"631T\",15,4,4,4,04,00,20,00*84956e00\n\tsystem status\tnormal 2 28.000000 0 0\trobot status\t343.177048\t30.494200\t11.842400\t0.569046\t-1.641285\t150.341250\t0.290000\t0.033000\n\t\n15:29:10.8\tlog_raw\tgps_raw\t#DUALANTENNAHEADINGA,USB3,0,47.5,FINESTEERING,2107,282568.800,02000000,d426,15824;SOL_COMPUTED,L1_FLOAT,-1.000000000,262.026367188,14.068168640,0.0,360.000000000,180.000000000,\"631T\",16,4,4,4,04,00,20,00*8f55d343\n\tsystem status\tnormal 2 28.000000 0 0\trobot status\t343.054788\t30.579973\t11.840500\t0.549366\t-1.618883\t150.501211\t0.308000\t-0.009000\n\t\n15:29:11.3\tlog_raw\tgps_raw\t#DUALANTENNAHEADINGA,USB3,0,50.0,FINESTEERING,2107,282569.300,02000000,d426,15824;SOL_COMPUTED,L1_FLOAT,-1.000000000,247.101364136,35.273887634,0.0,360.000000000,180.000000000,\"631T\",16,4,4,3,04,00,20,00*a64cde4f\n\tsystem status\tnormal 2 27.900000 0 0\trobot status\t342.933494\t30.664678\t11.838200\t0.752265\t-1.503616\t150.877739\t0.239000\t0.096000\n\t\n15:29:11.8\tlog_raw\tgps_raw\t#DUALANTENNAHEADINGA,USB3,0,50.0,FINESTEERING,2107,282569.800,02000000,d426,15824;SOL_COMPUTED,L1_FLOAT,-1.000000000,275.467193604,-13.373962402,0.0,360.000000000,180.000000000,\"631T\",15,4,4,4,04,00,20,00*431901e2\n\tsystem status\tnormal 2 27.800000 0 0\trobot status\t342.810357\t30.747828\t11.835100\t0.807077\t-1.414627\t151.385449\t0.350000\t-0.065000\n\t\n15:29:12.3\tlog_raw\tgps_raw\t#DUALANTENNAHEADINGA,USB3,0,51.0,FINESTEERING,2107,282570.300,02000000,d426,15824;SOL_COMPUTED,L1_FLOAT,-1.000000000,299.108795166,-43.822387695,0.0,360.000000000,180.000000000,\"631T\",15,4,4,4,04,00,20,00*983d1a38\n\tsystem status\tnormal 2 27.800000 0 0\trobot status\t342.689786\t30.827129\t11.831200\t0.757567\t-1.360819\t152.205755\t0.305000\t0.031000\n\t\n15:29:12.8\tlog_raw\tgps_raw\t#DUALANTENNAHEADINGA,USB3,0,51.0,FINESTEERING,2107,282570.800,02000000,d426,15824;SOL_COMPUTED,L1_FLOAT,-1.000000000,300.479248047,-46.014068604,0.0,360.000000000,180.000000000,\"631T\",16,4,4,4,04,00,20,00*471f7ae7\n\tsystem status\tnormal 2 27.700000 0 0\trobot status\t342.566147\t30.905173\t11.827000\t0.639719\t-1.500881\t153.184162\t0.317000\t0.011000\n\t\n15:29:13.3\tlog_raw\tgps_raw\t#DUALANTENNAHEADINGA,USB3,0,50.5,FINESTEERING,2107,282571.300,02000000,d426,15824;SOL_COMPUTED,L1_FLOAT,-1.000000000,281.970092773,-22.784423828,0.0,360.000000000,180.000000000,\"631T\",16,4,4,4,04,00,20,00*6e1b1745\n\tsystem status\tnormal 2 27.700000 0 0\trobot status\t342.441332\t30.981759\t11.823800\t0.444045\t-1.826412\t154.396160\t0.298000\t0.056000\n\t\n15:29:13.8\tlog_raw\tgps_raw\t#DUALANTENNAHEADINGA,USB3,0,50.5,FINESTEERING,2107,282571.800,02000000,d426,15824;SOL_COMPUTED,L1_FLOAT,-1.000000000,280.621307373,-20.287109375,0.0,360.000000000,180.000000000,\"631T\",17,4,4,4,04,00,20,00*f2e1552e\n\tsystem status\tnormal 2 27.700000 0 0\trobot status\t342.318103\t31.055550\t11.820900\t0.396277\t-1.911846\t155.620747\t0.308000\t0.054000\n\t\n15:29:14.3\tlog_raw\tgps_raw\t#DUALANTENNAHEADINGA,USB3,0,50.5,FINESTEERING,2107,282572.300,02000000,d426,15824;SOL_COMPUTED,L1_FLOAT,-1.000000000,248.617050171,42.773250580,0.0,360.000000000,180.000000000,\"631T\",14,4,4,4,04,00,20,00*4f7db08e\n\tsystem status\tnormal 2 27.700000 0 0\trobot status\t342.193438\t31.126975\t11.817000\t0.515418\t-1.918677\t156.785633\t0.307000\t0.033000\n\t\n15:29:14.8\tlog_raw\tgps_raw\t#DUALANTENNAHEADINGA,USB3,0,50.5,FINESTEERING,2107,282572.800,02000000,d426,15824;SOL_COMPUTED,L1_FLOAT,-1.000000000,246.696640015,43.920532227,0.0,360.000000000,180.000000000,\"631T\",15,4,4,4,04,00,20,00*5d650678\n\tsystem status\tnormal 2 27.700000 0 0\trobot status\t342.069284\t31.193916\t11.813400\t0.566601\t-1.873377\t157.924000\t0.288000\t0.031000\n\t\n15:29:15.3\tlog_raw\tgps_raw\t#DUALANTENNAHEADINGA,USB3,0,47.0,FINESTEERING,2107,282573.300,02000000,d426,15824;SOL_COMPUTED,L1_FLOAT,-1.000000000,245.228240967,45.089698792,0.0,360.000000000,180.000000000,\"631T\",15,6,6,6,04,00,20,20*cc0e41c2\n\tsystem status\tnormal 2 27.700000 0 0\trobot status\t341.943804\t31.257174\t11.809200\t0.577119\t-1.766781\t159.082306\t0.299000\t0.036000\n\t\n15:29:15.8\tlog_raw\tgps_raw\t#DUALANTENNAHEADINGA,USB3,0,47.0,FINESTEERING,2107,282573.800,02000000,d426,15824;SOL_COMPUTED,L1_FLOAT,-1.000000000,244.818725586,44.919303894,0.0,360.000000000,180.000000000,\"631T\",15,6,6,6,04,00,20,20*3059716a\n\tsystem status\tnormal 2 27.700000 0 0\trobot status\t341.816606\t31.317897\t11.806400\t0.535503\t-1.636626\t160.133846\t0.294000\t0.042000\n\t\n15:29:16.3\tlog_raw\tgps_raw\t#DUALANTENNAHEADINGA,USB3,0,50.0,FINESTEERING,2107,282574.300,02000000,d426,15824;SOL_COMPUTED,L1_FLOAT,-1.000000000,234.880477905,50.460414886,0.0,146.039688110,120.522598267,\"631T\",15,6,6,6,04,00,20,20*c87e4a6e\n\tsystem status\tnormal 2 27.800000 0 0\trobot status\t341.687565\t31.376397\t11.805300\t0.519008\t-1.590157\t161.111245\t0.302000\t0.027000\n\t\n15:29:16.8\tlog_raw\tgps_raw\t#DUALANTENNAHEADINGA,USB3,0,50.0,FINESTEERING,2107,282574.800,02000000,d426,15824;SOL_COMPUTED,L1_FLOAT,-1.000000000,234.896896362,50.646526337,0.0,146.141387939,119.189933777,\"631T\",17,6,6,6,04,00,20,20*6b091558\n\tsystem status\tnormal 2 27.700000 0 0\trobot status\t341.557954\t31.432292\t11.805500\t0.422846\t-1.540946\t162.074571\t0.285000\t0.034000\n\t\n15:29:17.3\tlog_raw\tgps_raw\t#DUALANTENNAHEADINGA,USB3,0,47.0,FINESTEERING,2107,282575.300,02000000,d426,15824;SOL_COMPUTED,L1_FLOAT,-1.000000000,247.052993774,4.654780388,0.0,360.000000000,180.000000000,\"631T\",15,6,6,6,04,00,20,20*6353fb30\n\tsystem status\tnormal 2 27.700000 0 0\trobot status\t341.428723\t31.486182\t11.803500\t0.517945\t-1.470910\t162.884549\t0.257000\t0.092000\n\t\n15:29:17.8\tlog_raw\tgps_raw\t#DUALANTENNAHEADINGA,USB3,0,47.0,FINESTEERING,2107,282575.800,02000000,d426,15824;SOL_COMPUTED,L1_FLOAT,-1.000000000,247.398025513,2.300915241,0.0,360.000000000,180.000000000,\"631T\",16,6,6,6,04,00,20,20*f5a4c1cb\n\tsystem status\tnormal 2 27.700000 0 0\trobot status\t341.295225\t31.539661\t11.799300\t0.725516\t-1.497623\t163.644133\t0.292000\t0.024000\n\t\n15:29:18.3\tlog_raw\tgps_raw\t\tsystem status\tnormal 2 27.800000 0 0\trobot status\t341.162657\t31.588802\t11.796600\t0.640006\t-1.565043\t164.356077\t0.288000\t0.031000\n\t\n15:29:18.8\tlog_raw\tgps_raw\t\tsystem status\tnormal 2 27.800000 0 0\trobot status\t341.028684\t31.637529\t11.794600\t0.568801\t-1.744057\t164.979933\t0.296000\t0.022000\n\t\n15:29:19.3\tlog_raw\tgps_raw\t#DUALANTENNAHEADINGA,USB3,0,49.5,FINESTEERING,2107,282577.300,02000000,d426,15824;SOL_COMPUTED,L1_FLOAT,-1.000000000,245.373901367,33.916652679,0.0,360.000000000,180.000000000,\"631T\",14,4,4,4,04,00,20,00*102f57bf\n\tsystem status\tnormal 2 27.900000 0 0\trobot status\t340.895392\t31.685711\t11.793900\t0.547011\t-1.826510\t165.564148\t0.286000\t0.047000\n\t\n15:29:19.8\tlog_raw\tgps_raw\t#DUALANTENNAHEADINGA,USB3,0,49.5,FINESTEERING,2107,282577.800,02000000,d426,15824;SOL_COMPUTED,L1_FLOAT,-1.000000000,248.600692749,29.202283859,0.0,360.000000000,180.000000000,\"631T\",15,4,4,3,04,00,20,00*eaef8a59\n\tsystem status\tnormal 2 27.800000 0 0\trobot status\t340.758690\t31.735475\t11.792600\t0.713412\t-1.928468\t166.025868\t0.246000\t0.103000\n\t\n15:29:20.3\tlog_raw\tgps_raw\t#DUALANTENNAHEADINGA,USB3,0,50.0,FINESTEERING,2107,282578.300,02000000,d426,15824;SOL_COMPUTED,L1_FLOAT,-1.000000000,273.737609863,2.134390354,0.0,360.000000000,180.000000000,\"631T\",15,4,4,4,04,00,20,00*8bcfc7c6\n\tsystem status\tnormal 2 27.800000 0 0\trobot status\t340.625924\t31.779494\t11.791300\t0.468461\t-1.855420\t166.462573\t0.313000\t0.000000\n\t\n15:29:20.8\tlog_raw\tgps_raw\t\tsystem status\tnormal 2 27.900000 0 0\trobot status\t340.493203\t31.821672\t11.788500\t0.231223\t-1.794056\t166.873260\t0.274000\t0.051000\n\t\n15:29:21.3\tlog_raw\tgps_raw\t#INSPVAXA,USB3,0,51.0,FINESTEERING,2107,282579.350,02000000,471d,15824;INS_ALIGNMENT_COMPLETE,INS_RTKFIXED,37.37041740707,126.72467743060,11.7862,22.3000,0.1031,-0.2921,-0.0179,0.173397794,-1.623675165,282.783174290,0.4573,0.2990,0.5534,0.1157,0.0933,0.0771,0.0996,0.1047,4.8395,0f000001,0*3f071db4\n\tsystem status\tnormal 2 27.900000 0 0\trobot status\t340.346899\t31.869021\t11.786200\t0.173398\t-1.623675\t167.216826\t0.226000\t0.113000\n\t\n15:29:21.8\tlog_raw\tgps_raw\t#DUALANTENNAHEADINGA,USB3,0,51.0,FINESTEERING,2107,282579.800,02000000,d426,15824;SOL_COMPUTED,L1_FLOAT,-1.000000000,253.552474976,36.318763733,0.0,360.000000000,180.000000000,\"631T\",12,4,4,4,04,00,20,00*83b3b49e\n\tsystem status\tnormal 2 27.900000 0 0\trobot status\t340.227718\t31.908242\t11.784900\t0.270794\t-1.547711\t167.577363\t0.263000\t0.048000\n\t\n15:29:22.3\tlog_raw\tgps_raw\t#DUALANTENNAHEADINGA,USB3,0,48.0,FINESTEERING,2107,282580.300,02000000,d426,15824;SOL_COMPUTED,L1_FLOAT,-1.000000000,276.287109375,16.184204102,0.0,360.000000000,180.000000000,\"631T\",13,4,4,4,04,00,20,00*58df2e4e\n\tsystem status\tnormal 2 27.900000 0 0\trobot status\t340.094651\t31.953158\t11.783700\t0.405495\t-1.591347\t167.909725\t0.269000\t0.048000\n\t\n15:29:22.8\tlog_raw\tgps_raw\t#INSPVAXA,USB3,0,48.0,FINESTEERING,2107,282580.850,02000000,471d,15824;INS_ALIGNMENT_COMPLETE,INS_RTKFIXED,37.37041861647,126.72467286120,11.7829,22.3000,0.1085,-0.2996,-0.0146,0.381599119,-1.778654518,281.769285798,0.4580,0.2991,0.5538,0.1158,0.0932,0.0771,0.0996,0.1049,4.8397,0f000001,0*ecbe1c22\n\tsystem status\tnormal 2 27.900000 0 0\trobot status\t339.942149\t32.003262\t11.782900\t0.381599\t-1.778655\t168.230714\t0.211000\t0.148000\n\t\n15:29:23.3\tlog_raw\tgps_raw\t\tsystem status\tnormal 2 27.900000 0 0\trobot status\t339.819525\t32.041971\t11.781400\t0.260429\t-1.799035\t168.510011\t0.307000\t0.001000\n\t\n15:29:23.8\tlog_raw\tgps_raw\t#DUALANTENNAHEADINGA,USB3,0,49.0,FINESTEERING,2107,282581.800,02000000,d426,15824;SOL_COMPUTED,L1_FLOAT,-1.000000000,244.951904297,46.151142120,0.0,329.327331543,180.000000000,\"631T\",12,4,4,4,04,00,20,00*1c1834ad\n\tsystem status\tnormal 2 27.900000 0 0\trobot status\t339.683616\t32.084123\t11.778500\t0.213215\t-1.826145\t168.834854\t0.257000\t0.063000\n\t\n15:29:24.3\tlog_raw\tgps_raw\t\tsystem status\tnormal 2 27.900000 0 0\trobot status\t339.548246\t32.126267\t11.775900\t0.236515\t-1.715051\t169.175040\t0.422000\t-0.161000\n\t\n15:29:24.8\tlog_raw\tgps_raw\t#INSPVAXA,USB3,0,49.5,FINESTEERING,2107,282582.850,02000000,471d,15824;INS_ALIGNMENT_COMPLETE,INS_RTKFIXED,37.37042013529,126.72466675412,
